vi "PH_Timing.contents.vi"   [LabVIEW 2014, in "PH_Timing.lvlib"]
doc: "This class is forseen to control all time related instances, mainly all gate and delay generators of PHELIX.\n\nThis class is part of the PHELIX application layer."
uses:
  PH_Timing.lvlib
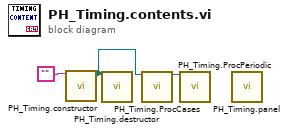
[diagram p0: block diagram]
diagram:
  n1 = call "PH_Timing.constructor.vi"("name"="") -> ("i ref out"=w1:refnum<vi>)  [unwired: 16 in, 2 out]
  n2 = call "PH_Timing.destructor.vi"("i ref in"=w1) -> ()  [unwired: 18 in, 1 out]
  n3 = call "PH_Timing.ProcCases.vi"("i ref in"=w1) -> ("i ref out"=w3:refnum<vi>)  [unwired: 16 in, 2 out]
  n4 = call "PH_Timing.ProcPeriodic.vi"("i ref in"=w3) -> ()  [unwired: 16 in, 3 out]
  n5 = call "PH_Timing.panel.vi"() -> ()  [unwired: 19 in, 1 out]
